vi "runSalMonitor.vi"(8 "error in (no error)":errorcluster, 9 "pathOfOutput":path, 10 "pathOfSalMonitor":path, 11 "TestProcess in":refnum<class "TestProcess.lvclass">) -> (0 "error out":errorcluster, 3 "TestProcess out":refnum<class "TestProcess.lvclass">)   [LabVIEW 2018, in "TestProcess.lvclass"]
doc: "Run the SAL monitor in the background."
uses:
  TestProcess.lvclass
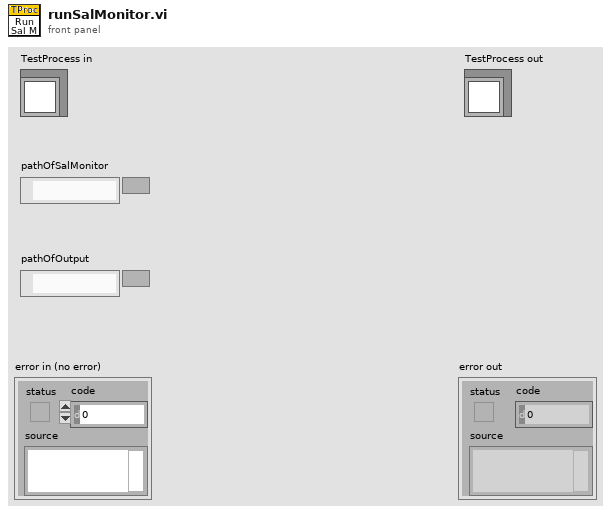
[diagram p1: front panel]
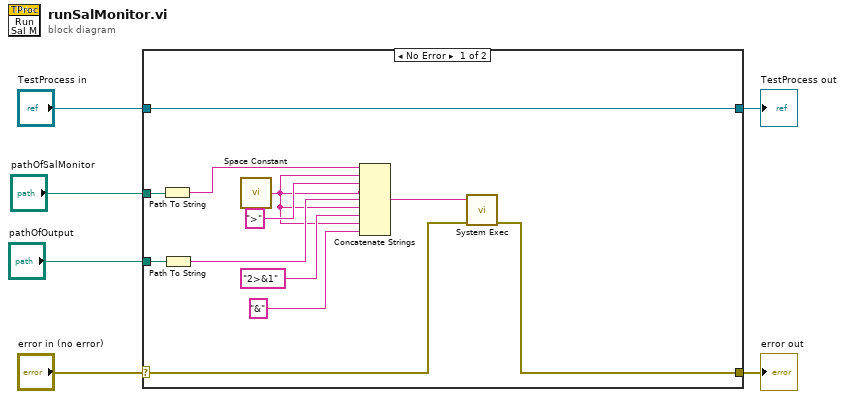
[diagram p0: block diagram]
diagram:
  n1 = case shown="No Error" "error in (no error)" {
    selector: "error in (no error)" -> [w16 w20]
    tunnel: [w15 w20] -> w5
    tunnel: [w18 w19] -> w3
    tunnel: "TestProcess in" -> [w18 w19]
    tunnel: "pathOfSalMonitor" -> [w17 _]
    tunnel: "pathOfOutput" -> [w14 _]
    frame No Error {
      n2 = Path To String(path=w17) -> (string=w7:string)
      n3 = Path To String(path=w14) -> (string=w12:string)
      n4 = call <vilib>:"Space Constant.vi"() -> ("String"=w10:string)
      n5 = Concatenate Strings(w7, w10, ">", w10, w12, w10, "2>&1", w10, "&") -> (w8:string)
      n6 = call <vilib>:"System Exec.vi"("error in (no error)"=w16, "command line"=w8) -> ("error out"=w15:errorcluster)  [unwired: 6 in, 3 out]
    }
    frame Error {
    }
  }
  "error out" <- w5
  "TestProcess out" <- w3
